vi "Launch as Nested.vi"(4 "Disable Events (F)":bool, 5 "GUI Info (Default)":T1={"Color"=4547941, "Name"=""}, 6 "Auto Apply (T)":bool=TRUE, 7 "Register (T)":bool=TRUE, 8 "error in (no error)":errorcluster, 10 "GUI":refnum<vi>, 11 "Parent in":refnum<class "Module.lvclass">) -> (0 "error out":errorcluster, 2 "MessageQ":refnum<class "MessageQ.lvclass">, 3 "Parent":refnum<class "Module.lvclass">)   [LabVIEW 2020, in "VolatusGUI.lvlib" / "GUI Helper.lvclass"]
uses:
  GUI Helper.lvclass
  Volatus/Module/Module.lvclass
  Volatus/MessageQ/MessageQ.lvclass
  C:/dev/lv20CE/relink/lv-volatus/Volatus/Module/Module.lvclass
  VolatusConfig/VolatusConfigElement/VolatusConfigElement.lvclass
  GUI Helper.lvclass/GUI Helper.ctl
  C:/dev/lv20CE/relink/lv-volatus/VolatusGUI/GUI Helper/GUI Helper.lvclass
  GUI Info.ctl
  VolatusGUI.lvlib
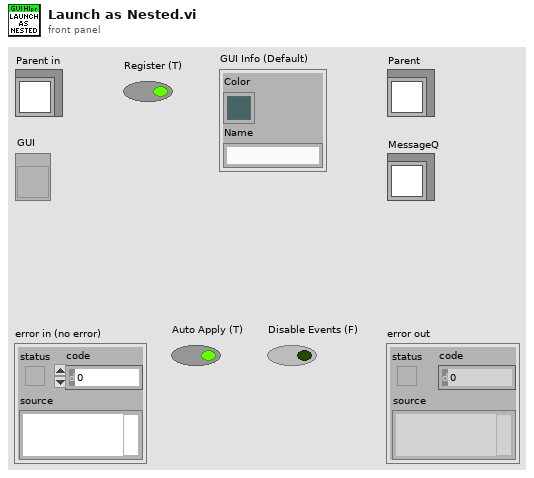
[diagram p1: front panel]
types:
  T1 = typedef "VolatusGUI.lvlib/GUI Info.ctl" = cluster{"Color":u32, "Name":string}
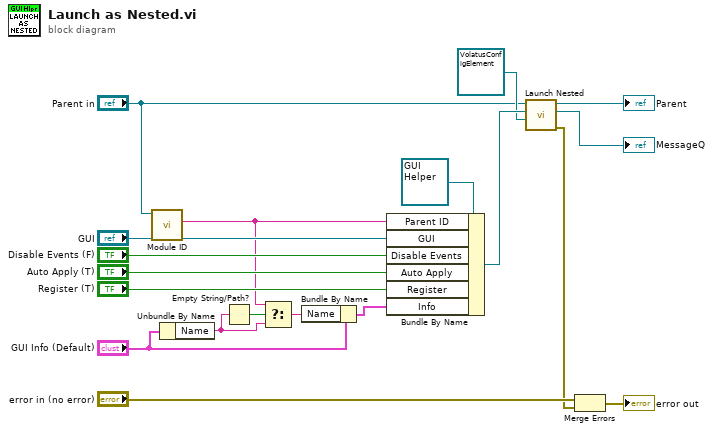
[diagram p0: block diagram]
diagram:
  n1 = call-dynamic "Module ID.vi"("Module in"="Parent in") -> ("Module ID"=w4:string)  [unwired: 10 in]
  n2 = Unbundle By Name("GUI Info (Default)") -> ("Name"=w5:string)
  n3 = Empty String/Path?(string/path=w5) -> (empty?=w6:bool)
  n4 = Select(t=w4, s=w6, f=w5) -> (s? t:f=w2:string)
  n5 = Bundle By Name(cluster="GUI Info (Default)", "Name"=w2) -> (w1:T1)
  n6 = Bundle By Name(cluster=refnum<class "GUI Helper.lvclass"> refnum ("GUI Helper in"), "Parent ID"=w4, "GUI"="GUI", "Disable Events"="Disable Events (F)", "Auto Apply"="Auto Apply (T)", "Register"="Register (T)", "Info"=w1) -> (w16:refnum<class "GUI Helper.lvclass">)
  n7 = call "Launch Nested.vi"("Config Element"=refnum<class "VolatusConfigElement.lvclass"> refnum, "Nested Module"=w16, "Parent in"="Parent in") -> ("error out"=w10:errorcluster, "MessageQ"=→"MessageQ":refnum<class "MessageQ.lvclass">, "Parent out"=→"Parent":refnum<class "Module.lvclass">)  [unwired: 6 in]
  n8 = Merge Errors("error in (no error)", w10) -> (→"error out":errorcluster)
